vi "Bar Plot.vi"() -> ()   [LabVIEW 2013]
uses:
  <vilib>/Heliosphere Research LLC/Advanced Plotting Toolkit/properties/Line.ctl
  <vilib>/Heliosphere Research LLC/Advanced Plotting Toolkit/properties/Line_Style.ctl
  <vilib>/Heliosphere Research LLC/Advanced Plotting Toolkit/typedefs/PlotColor.ctl
  <vilib>/Heliosphere Research LLC/Advanced Plotting Toolkit/api_plotting/BarProperties.ctl
  <vilib>/Heliosphere Research LLC/Advanced Plotting Toolkit/properties/Display.ctl
  <vilib>/Heliosphere Research LLC/Advanced Plotting Toolkit/Advanced Plotting Toolkit.lvlib
panel:
  in  "\"Snow\" Bar Color":u32(colorbox)=11579568
  in  "\"Rain\" Bar Color":u32(colorbox)=3381759
  in  "Bar Outlines":T1={"Style"=enum."Automatic", "Color"=2147483647, "Width"=nan} {"Color" items=["Automatic"=2147483647, "Black"=0, "White"=16777215, "Red"=16711680, "Green"=2263842, "Blue"=255, "Cyan"=65535, "Magenta"=16711935, "Yellow"=16776960]}
  out "Stacked Bar Plot":picture
  # "Bar Plot"
  # "This example demonstrates a simple bar plot, along with some\nspecial features like bar stacking and tick relabeling.\n\nBar plots consist of a series of rectangles; the only required\ninput is the rectangle heights.  In this example, two populations\nof data are displayed: daily precipitation totals for rain and\nsnow.\n\nUsing the optional Bar Bottoms terminal, the Rain bars start\nat the top of the Snow bars, making a stacked bar plot.\n\nThe appearance of the bars can also be changed.  Here we\nmanually pick colors for the bars; otherwise, they will use the\nautomatic color cycle."
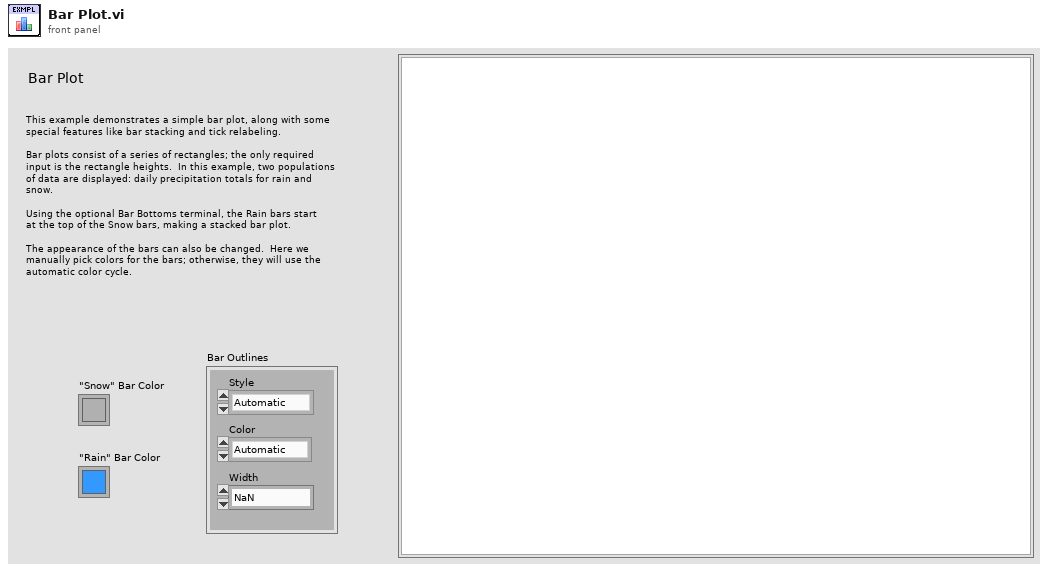
[diagram p1: front panel]
types:
  T1 = typedef "Advanced Plotting Toolkit.lvlib/Line.ctl" = cluster{"Style":T2, "Color":T3, "Width":sgl}
  T2 = typedef "Advanced Plotting Toolkit.lvlib/Line_Style.ctl" = enum16{"Automatic", "Solid", "Dashed", "Dotted", "Dash-dot", "Invisible"}
  T3 = typedef "Advanced Plotting Toolkit.lvlib/PlotColor.ctl" = u32
  T4 = typedef "Advanced Plotting Toolkit.lvlib/BarProperties.ctl" = cluster{"Bar Color":T3, "Line":T1, "Display":T5}
  T5 = typedef "Advanced Plotting Toolkit.lvlib/Display.ctl" = cluster{"Alpha":dbl, "Z Order":dbl}
  T6 = typedef "Advanced Plotting Toolkit.lvlib/PlotID.ctl" = i32
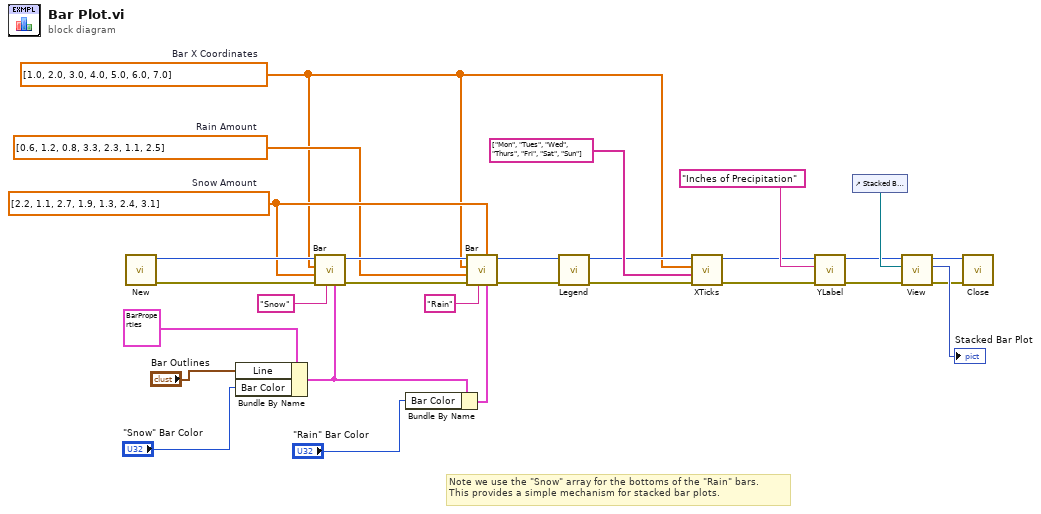
[diagram p0: block diagram]
diagram:
  w21 = dbl[] [0.6, 1.2, 0.8, 3.3, 2.3, 1.1, 2.5]  # Rain Amount
  w22 = dbl[] [2.2, 1.1, 2.7, 1.9, 1.3, 2.4, 3.1]  # Snow Amount
  w3 = dbl[] [1.0, 2.0, 3.0, 4.0, 5.0, 6.0, 7.0]  # Bar X Coordinates
  # "Note we use the \"Snow\" array for the bottoms of the \"Rain\" bars.\nThis provides a simple mechanism for stacked bar plots."
  n1 = call <vilib>:"New.vi"() -> ("error out"=w26:errorcluster, "Plot ID"=w27:T6)  [unwired: 10 in]
  n2 = Bundle By Name(cluster=T4 {"Bar Color"=2147483647, "Line"={"Style"=enum."Automatic", "Color"=2147483647, "Width"=nan}, "Display"={"Alpha"=nan, "Z Order"=nan}} ("Bar Plot Properties"), "Line"="Bar Outlines", "Bar Color"="\"Snow\" Bar Color") -> (w9:T4)
  n3 = call <vilib>:"Bar.vi"("Properties"=w9, "Legend Title"="Snow", "error in (no error)"=w26, "Bar Lengths"=w22, "X Coordinates"=w3, "Plot ID"=w27) -> ("error out"=w23:errorcluster, "Plot ID Out"=w24:T6)  [unwired: 4 in]
  n4 = Bundle By Name(cluster=w9, "Bar Color"="\"Rain\" Bar Color") -> (w8:T4)
  n5 = call <vilib>:"Bar.vi"("Properties"=w8, "Bar Bottoms"=w22, "Legend Title"="Rain", "error in (no error)"=w23, "Bar Lengths"=w21, "X Coordinates"=w3, "Plot ID"=w24) -> ("error out"=w19:errorcluster, "Plot ID Out"=w20:T6)  [unwired: 3 in]
  n6 = call <vilib>:"Legend.vi"("error in (no error)"=w19, "Plot ID"=w20) -> ("error out"=w16:errorcluster, "Plot ID Out"=w17:T6)  [unwired: 8 in]
  n7 = call <vilib>:"XTicks.vi"("error in (no error)"=w16, "Tick Labels"=string[] ["Mon", "Tues", "Wed", "Thurs", "Fri", "Sat", "Sun"], "Tick Locations"=w3, "Plot ID"=w17) -> ("error out"=w5:errorcluster, "Plot ID Out"=w6:T6)  [unwired: 6 in]
  n8 = call <vilib>:"YLabel.vi"("error in (no error)"=w5, "Label"="Inches of Precipitation", "Plot ID"=w6) -> ("error out"=w14:errorcluster, "Plot ID out"=w15:T6)  [unwired: 7 in]
  n9 = control-ref of="Stacked Bar Plot"() -> (w28:refnum<vi>)
  n10 = call <vilib>:"View.vi"("error in (no error)"=w14, "Ref for Sizing"=w28, "Plot ID"=w15) -> ("error out"=w1:errorcluster, "Picture"=→"Stacked Bar Plot":picture, "Plot ID Out"=w25:T6)  [unwired: 6 in]
  n11 = call <vilib>:"Close.vi"("error in (no error)"=w1, "Plot ID"=w25) -> ()  [unwired: 9 in, 1 out]
